vi "Parse Board Setup.vi"(8 "error in":errorcluster, 11 "node in":refnum<k20>) -> (0 "error out":errorcluster, 2 "portSetup":T1 {"portConfig" items=["FDX_SINGLE", "FDX_REDUNDANT"]; "portSpeed" items=["FDX_100MBIT", "FDX_10MBIT", "FDX_AUTO_100MBIT", "FDX_AUTO_10MBIT", "FDX_AUTO_ERROR", "FDX_1000MBIT"]}, 3 "node out":refnum<k20>)   [LabVIEW 2020, in "AIM ARINC 664 Import.lvlib"]
uses:
  AIM ARINC 664 Import.lvlib
  _typedefs/board_setup.ctl
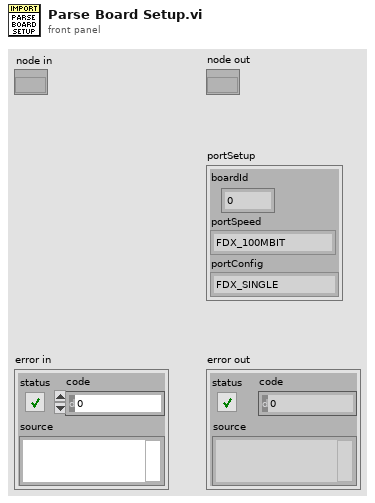
[diagram p1: front panel]
types:
  T1 = typedef "AIM ARINC 664 Import.lvlib/board_setup.ctl" = cluster{"boardId":u32, "portSpeed":u32, "portConfig":u32}
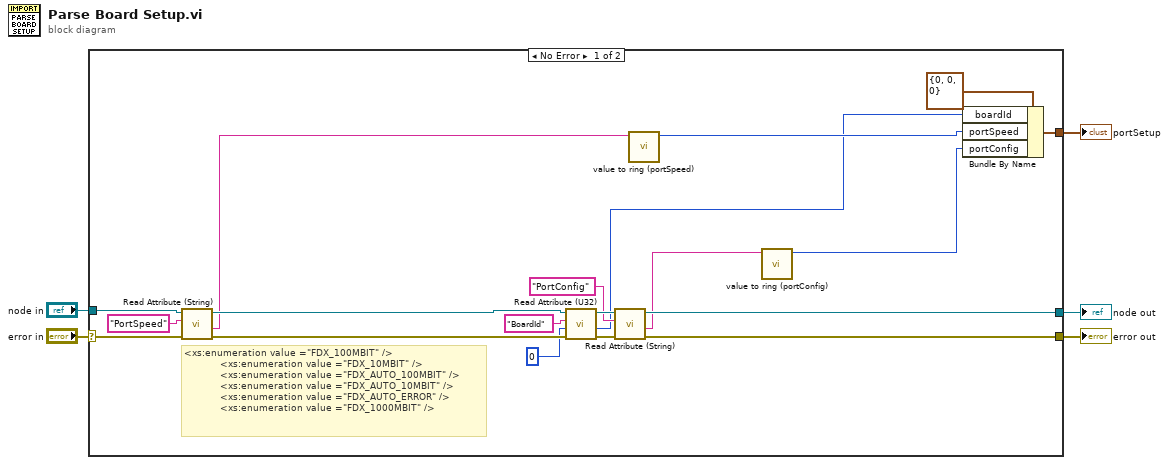
[diagram p0: block diagram]
diagram:
  n1 = case shown="No Error" "error in" {
    selector: "error in" -> [w15 w26]
    tunnel: "node in" -> [w20 w25]
    tunnel: [w9 w26] -> w4
    tunnel: [w24 _] -> w1
    tunnel: [w19 w25] -> w2
    frame No Error {
      # "<xs:enumeration value =\"FDX_100MBIT\" />\n            <xs:enumeration value =\"FDX_10MBIT\" />\n            <xs:enumeration value =\"FDX_AUTO_100MBIT\" />\n            <xs:enumeration value =\"FDX_AUTO_10MBIT\" />\n            <xs:enumeration value =\"FDX_AUTO_ERROR\" />\n            <xs:enumeration value =\"FDX_1000MBIT\" />"
      n2 = call "Read Attribute (String).vi"("error in"=w15, "Attribute Name"="PortSpeed" ("Tag Name"), "node in"=w20) -> ("error out"=w13:errorcluster, "value"=w14:string, "node out"=w18:refnum<k20>)  [unwired: 6 in]
      n3 = call "Read Attribute (U32).vi"("error in"=w13, "default"=u32 0, "Attribute Name"="BoardId" ("Tag Name"), "node in"=w18) -> ("error out"=w10:errorcluster, "value"=w7:u32, "node out"=w17:refnum<k20>)  [unwired: 5 in]
      n4 = call "Read Attribute (String).vi"("error in"=w10, "Attribute Name"="PortConfig" ("Tag Name"), "node in"=w17) -> ("error out"=w9:errorcluster, "value"=w8:string, "node out"=w19:refnum<k20>)  [unwired: 6 in]
      n5 = call "value to ring (portSpeed).vi"("value"=w14) -> ("portSpeed"=w22:u32)  [unwired: 10 in]
      n6 = call "value to ring (portConfig).vi"("value"=w8) -> ("portConfig"=w21:u32)  [unwired: 10 in]
      n7 = Bundle By Name(cluster=T1 {"boardId"=0, "portSpeed"=0, "portConfig"=0} ("portSetup"), "boardId"=w7, "portSpeed"=w22, "portConfig"=w21) -> (w24:T1)
    }
    frame Error {
    }
  }
  "error out" <- w4
  "node out" <- w2
  "portSetup" <- w1
